vi "Integrator Start-Stop.vi"(8 "error in (no error)":errorcluster, 9 "Start/Stop (F: Stop)":bool, 10 "Element (All: 0)":T1(ring), 11 "Yokogawa WT2X0 in":refnum<class "Yokogawa WT2X0.lvclass">) -> (0 "error out":errorcluster, 2 "VISA session":refnum<visa-resource-name>, 3 "Yokogawa WT2X0 out":refnum<class "Yokogawa WT2X0.lvclass">)   [LabVIEW 2013, in "Generic Power Analyzer.lvlib" / "Yokogawa WT2X0.lvlib" / "Yokogawa WT2X0.lvclass"]
uses:
  Yokogawa WT2X0.lvclass
  Generic Power Analyzer/Generic Power Analyzer.lvclass
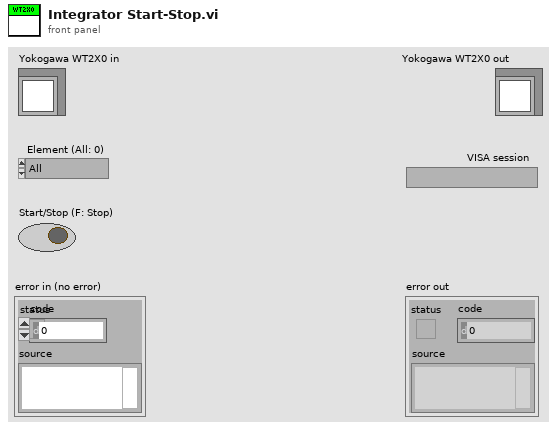
[diagram p1: front panel]
types:
  T1 = enum16{"All", "Element 1", "Element 2", "Element 3", "Element 4", "Element 5", "Element 6"}
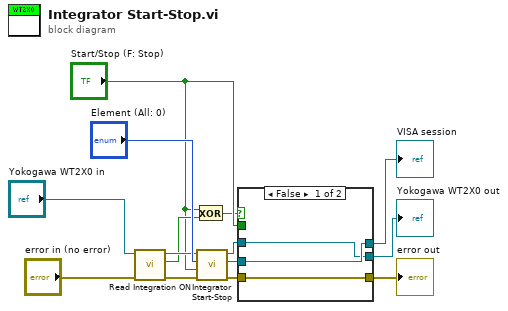
[diagram p0: block diagram]
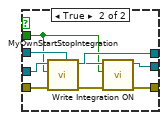
[diagram p2: hidden frame]
diagram:
  n1 = call-dynamic "Read Integration ON.vi"("error in (no error)"="error in (no error)", "Yokogawa WT2X0 in"="Yokogawa WT2X0 in") -> ("error out"=w6:errorcluster, "Integration ON"=w5:bool, "Yokogawa WT2X0 out"=w8:refnum<class "Yokogawa WT2X0.lvclass">)  [unwired: 7 in]
  n2 = Exclusive Or(1:w5, 2:"Start/Stop (F: Stop)") -> (0:w3:bool)
  n3 = call-parent "Integrator Start-Stop.vi"("error in (no error)"=w6, "Start/Stop (F: Stop)"="Start/Stop (F: Stop)", "Element (All: 0)"="Element (All: 0)", "Universal Power Meter in"=w8) -> ("error out"=w10:errorcluster, "VISA session"=w13:refnum<visa-resource-name>, "Universal Power Meter out"=w2:refnum<class "Universal Power Meter.lvclass">)  [unwired: 5 in]
  n4 = case shown="False" w3 {
    tunnel: w13 -> [w17 w25]
    tunnel: [w16 w19] -> w12
    tunnel: [w17 w24] -> w11
    tunnel: w10 -> [w16 w23]
    tunnel: "Start/Stop (F: Stop)" -> [_ w18]
    tunnel: w2 -> [w15 w22]
    tunnel: [w15 w21] -> w1
    frame False {
    }
    frame True {
      n5 = call "MyOwnStartStopIntegration.vi"("Error In"=w23, "Start/Stop"=w18, "VISA resource name"=w25) -> ("Error Out"=w20:errorcluster, "VISA resource name 2"=w24:refnum<visa-resource-name>)  [unwired: 7 in]
      n6 = call-dynamic "Write Integration ON.vi"("error in (no error)"=w20, "Integration ON"=w18, "Yokogawa WT2X0 in"=w22) -> ("error out"=w19:errorcluster, "Yokogawa WT2X0 out"=w21:refnum<class "Yokogawa WT2X0.lvclass">)  [unwired: 7 in]
    }
  }
  "error out" <- w12
  "Yokogawa WT2X0 out" <- w1
  "VISA session" <- w11
